vi "receiver_6.vi"() -> ()   [LabVIEW 2022 SP3]
uses:
  <vilib>/addons/Modulation/Analog/support/mod_Set Error Source.vi
  <vilib>/addons/Modulation/Digital/Support/Common/Validators/mod_Generate Filter Coefficients Validate.vi
  <vilib>/addons/Modulation/Digital/General/subVIs/mod_Generate Filter Coefficients.vi
  <instrlib>/niUSRP/niUSRP Fetch Rx Data (CDB Cluster).vi
  <vilib>/addons/Modulation/Digital/General/MT Generate QAM System Parameters(M).vi
  <vilib>/addons/Modulation/niDMT.lvlib
panel:
  in  "stop 2":bool
  in  "gain":dbl format="%#_6f"
  in  "IQ rate":dbl=100000.0 format="%#_6p"
  in  "active antenna":string
  in  "carrier frequency":dbl=100000.0 format="%#_6p"
  in  "device names":refnum<k15>
  in  "filter parameter":dbl=0.5 format="%.2f"
  out "Received":T1(graph)
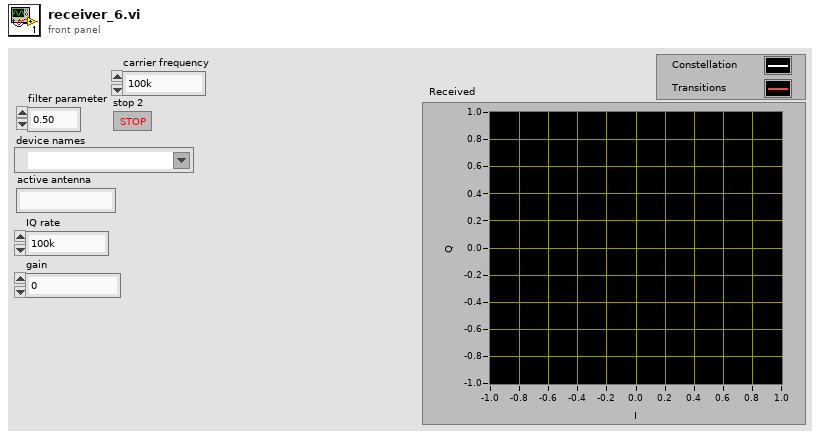
[diagram p1: front panel]
types:
  T1 = cluster{"Decimated Array":dbl[], "Decimated Array":dbl[]}[]
  T2 = enum16{"FSK", "PSK", "QAM", "MSK", "PAM", "ASK", "CPM"}
  T3 = enum16{"none", "Raised Cosine", "Root Raised Cos", "Gaussian"}
  T4 = cluster{"samples per symbol (16)":i32, "symbol map":cdb[]}
  T5 = typedef "niAMT.lvlib/Complex Data Waveform.ctl" = cluster{"t0":dbl, "dt":dbl, "Y":cdb[]}
  T6 = cluster{"constellation":dbl[], "oversampled data":dbl[]}[]
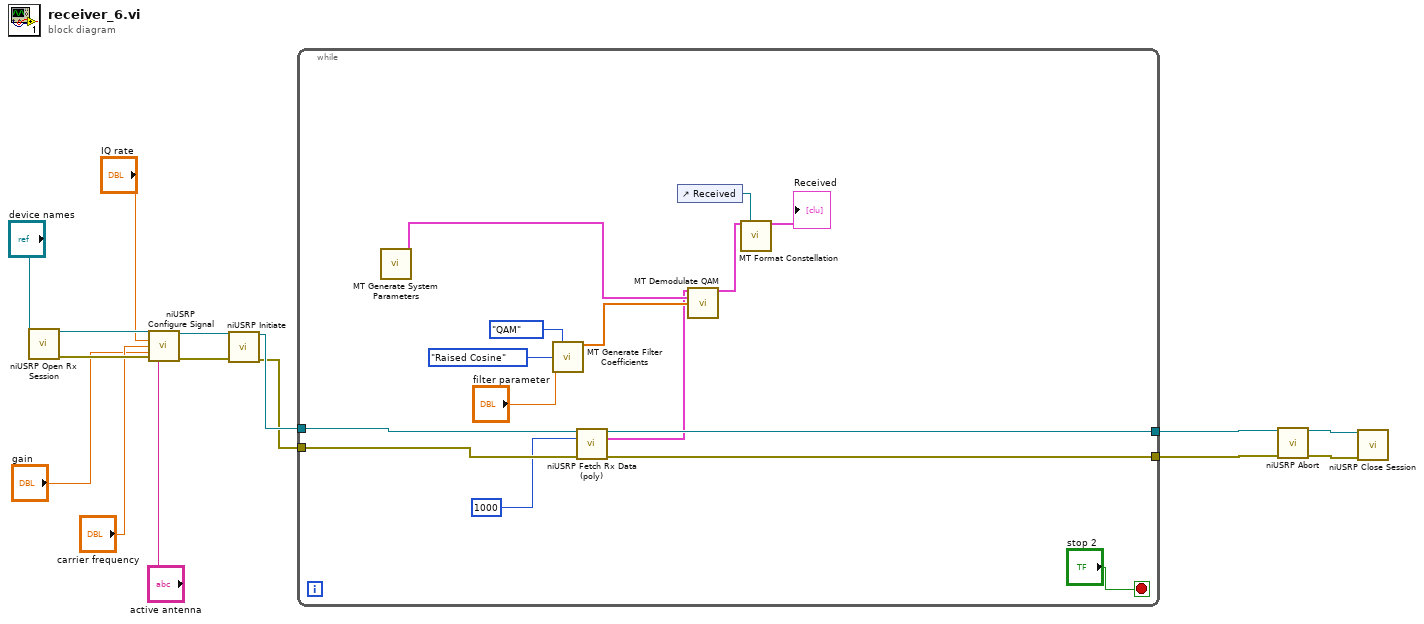
[diagram p0: block diagram]
diagram:
  n1 = call <instrlib>:"niUSRP Open Rx Session.vi"("device names"="device names") -> ("session handle out"=w15:refnum<k15>, "error out"=w14:errorcluster)  [unwired: 13 in]
  n2 = call <instrlib>:"niUSRP Configure Signal.vi"("session handle"=w15, "IQ rate"="IQ rate", "carrier frequency"="carrier frequency", "gain"="gain", "error in (no error)"=w14, "active antenna"="active antenna") -> ("session handle out"=w13:refnum<k15>, "error out"=w12:errorcluster)  [unwired: 5 in, 3 out]
  n3 = call <instrlib>:"niUSRP Initiate.vi"("session handle"=w13, "error in (no error)"=w12) -> ("session handle out"=w11:refnum<k15>, "error out"=w10:errorcluster)  [unwired: 12 in]
  n4 = while {
    tunnel: w11 -> [w23]
    tunnel: w10 -> [w22]
    tunnel: [w21] -> w9
    tunnel: [w20] -> w6
    stop <- "stop 2" stop-if-true
    n5 = call-poly <vilib>:"MT Generate System Parameters.vi"() -> ("QAM system parameters"=w19:T4)  [unwired: 13 in, 2 out]
    n6 = call <vilib>:"MT Generate Filter Coefficients.vi"("pulse shaping filter (none)"=T3."Raised Cosine", "modulation type"=T2."QAM", "filter parameter"="filter parameter") -> ("pulse shaping filter coefficients"=w30:dbl[])  [unwired: 10 in, 2 out]
    n7 = call-poly <instrlib>:"niUSRP Fetch Rx Data (poly).vi"("session handle"=w23, "number of samples"=i64 1000, "error in (no error)"=w22) -> ("session handle out"=w21:refnum<k15>, "data"=w18:cluster{"t0":dbl, "dt":dbl, "Y":cdb[]}, "error out"=w20:errorcluster)  [unwired: 9 in, 1 out]
    n8 = control-ref of="Received"() -> (w28:refnum<vi>)
    n9 = call <vilib>:"MT Demodulate QAM.vi"("input complex waveform"=w18, "QAM system parameters"=w19, "matched filter coefficients"=w30) -> ("recovered complex waveform"=w27:T5)  [unwired: 8 in, 4 out]
    n10 = call <vilib>:"MT Format Constellation.vi"("waveform"=w27, "constellation reference"=w28) -> ("constellation graph"=→"Received":T6)  [unwired: 3 in, 10 out]
  }
  n11 = call <instrlib>:"niUSRP Abort.vi"("session handle"=w9, "error in (no error)"=w6) -> ("session handle out"=w8:refnum<k15>, "error out"=w7:errorcluster)  [unwired: 12 in]
  n12 = call <instrlib>:"niUSRP Close Session.vi"("session handle"=w8, "error in (no error)"=w7) -> ()  [unwired: 13 in, 1 out]
